vi "XML Parse String.vi"(3 "Attribut Name":string, 7 "XML Response":string) -> (0 "Wert-String":string, 2 "XML Response gekürzt":string)   [LabVIEW 2020, in "FT-IR.lvlib" / "TOOLweb Interface.lvlib" / "TOOLweb Interface Hilfs-VIs.lvlib"]
doc: "Sucht in dem XML-Poll-Response-String \"XML-Response\" den Eintrag mit dem Elementnamen \"Attribut Name\" und liefert dessen Wert in \"Wert-String\". \n\nDer Eintrag wird dann entfernt, damit eine weiteres Parser-VI am Ausgang \"XML Response gekürzt\" nicht wieder den ganzen String durchsuchen muss."
uses:
  TOOLweb Interface Hilfs-VIs.lvlib
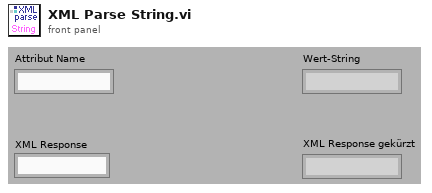
[diagram p1: front panel]
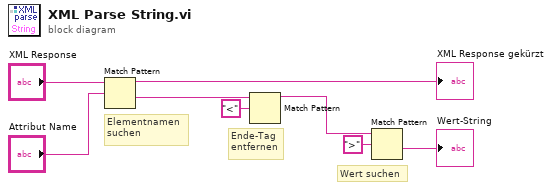
[diagram p0: block diagram]
diagram:
  # "Wert suchen"
  # "Elementnamen\nsuchen"
  # "Ende-Tag\nentfernen"
  n1 = Match Pattern(string="XML Response", regular expression="Attribut Name") -> (before substring=→"XML Response gekürzt":string, after substring=w6:string)  [unwired: 3 out]
  n2 = Match Pattern(string=w6, regular expression="<" ("Regulärer Ausdruck")) -> (before substring=w3:string)  [unwired: 4 out]
  n3 = Match Pattern(string=w3, regular expression=">" ("Regulärer Ausdruck")) -> (after substring=→"Wert-String":string)  [unwired: 4 out]
